vi "ProcAutoScan.vi"(2 "Body":u8[](array[numeric]), 3 "Length":u16) -> (0 "AutoScan Data":dbl format="%.2f", 1 "Error":u32)   [LabVIEW 2016]
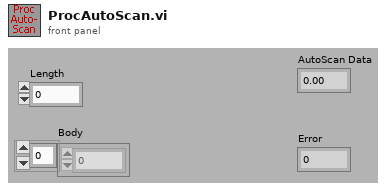
[diagram p1: front panel]
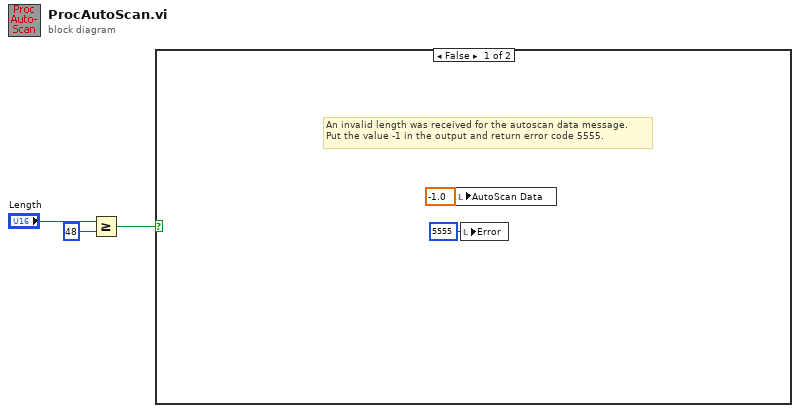
[diagram p0: block diagram]
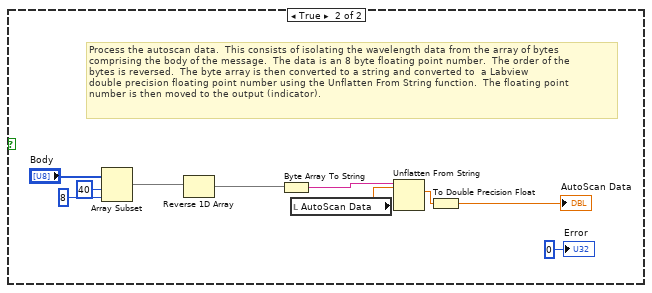
[diagram p2: hidden frame]
diagram:
  n1 = Greater Or Equal?(x="Length", y=u16 48) -> (x >= y?=w1:bool)
  n2 = case shown="False" w1 {
    frame False {
      # "An invalid length was received for the autoscan data message.\nPut the value -1 in the output and return error code 5555."
      n3 = local write "AutoScan Data"(-1.0 ("AutoScan Data")) -> ()
      n4 = local write "Error"(u32 5555 ("Error")) -> ()
    }
    frame True {
      # "Process the autoscan data.  This consists of isolating the wavelength data from the array of bytes\ncomprising the body of the message.  The data is an 8 byte floating point number.  The order of the\nbytes is reversed.  The byte array is then converted to a string and converted to  a Labview\ndouble precision floating point number using the Unflatten From String function.  The floating point\nnumber is then moved to the output (indicator)."
      n5 = Array Subset "Array Subset"(array="Body", index=40 ("Array Index"), length=8 ("Array Length")) -> (w8:u8[])
      n6 = Reverse 1D Array(array=w8) -> (reversed array=w7:u8[])
      n7 = Byte Array To String(unsigned byte array=w7) -> (string=w13:string)
      n8 = local read "AutoScan Data"() -> (w12:dbl)
      n9 = Unflatten From String(type=w12, binary string=w13) -> (value=w14:dbl)  [unwired: 3 in, 2 out]
      n10 = To Double Precision Float(number=w14) -> (double precision float=→"AutoScan Data":dbl)
      "Error" <- u32 0 ("Error")
    }
  }
